vi "Example Loopback - Read Callback.vi"(4 "Read":refnum<user-event>, 5 "Event Data":cluster{"sender":refnum<k24>, "message":u16[]}, 6 "Control Ref":refnum<k24>, 7 "Event Common Data":T1) -> ()   [LabVIEW 2013]
uses:
  C:/tf/play/labview/Tinkerforge.dll
  Tinkerforge.dll
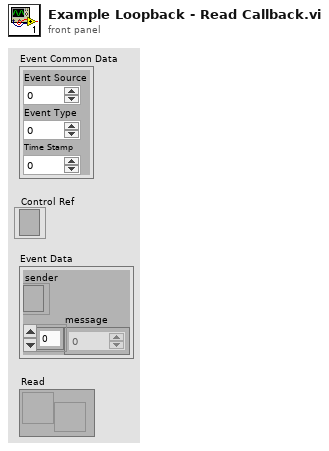
[diagram p1: front panel]
types:
  T1 = cluster{"Event Source":i32, "Event Type":u32, "Time Stamp":u32}
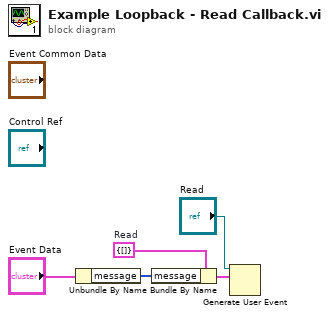
[diagram p0: block diagram]
diagram:
  w4 = cluster{"message":u16[]} {"message"=[]}  # Read
  n1 = Unbundle By Name("Event Data") -> ("message"=w3:u16[])
  n2 = Bundle By Name(cluster=w4, "message"=w3) -> (w1:cluster{"message":u16[]})
  n3 = Generate User Event(user event="Read", event data cluster=w1) -> ()  [unwired: 2 in, 2 out]
